vi "RDS Child Subscription.vi"(8 "error in (no error)":errorcluster, 11 "AIP Instrument in":refnum<class "AIP Instrument.lvclass">) -> (0 "error out":errorcluster, 2 "Subscribed IDs":T1[](array[typedef]), 3 "AIP Instrument out":refnum<class "AIP Instrument.lvclass">)   [LabVIEW 2015]
uses:
  Libraries/RDS Framework/RDS Message ID.ctl
  Libraries/RDS Framework/RDS Framework.lvlib
  Actors/RDS Parent Actor/RDS Parent Actor/RDS Parent Actor.lvclass
  AIP Instrument.lvclass
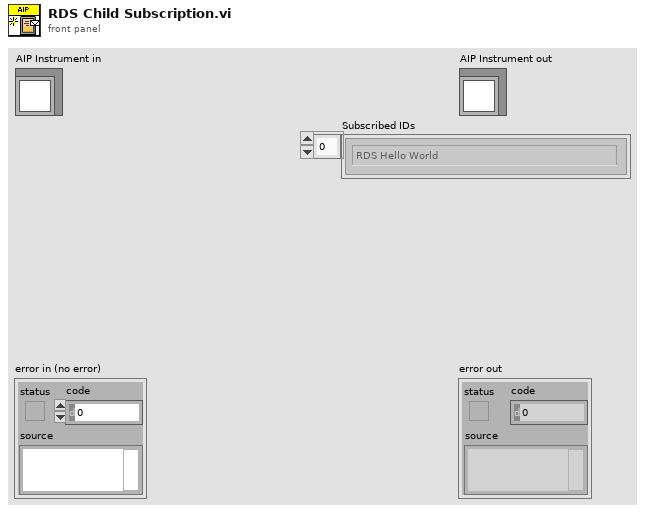
[diagram p1: front panel]
types:
  T1 = typedef "RDS Framework.lvlib/RDS Message ID.ctl" = enum16{"RDS Hello World", "String Message", "AIP_Status", "AIP_Command"}
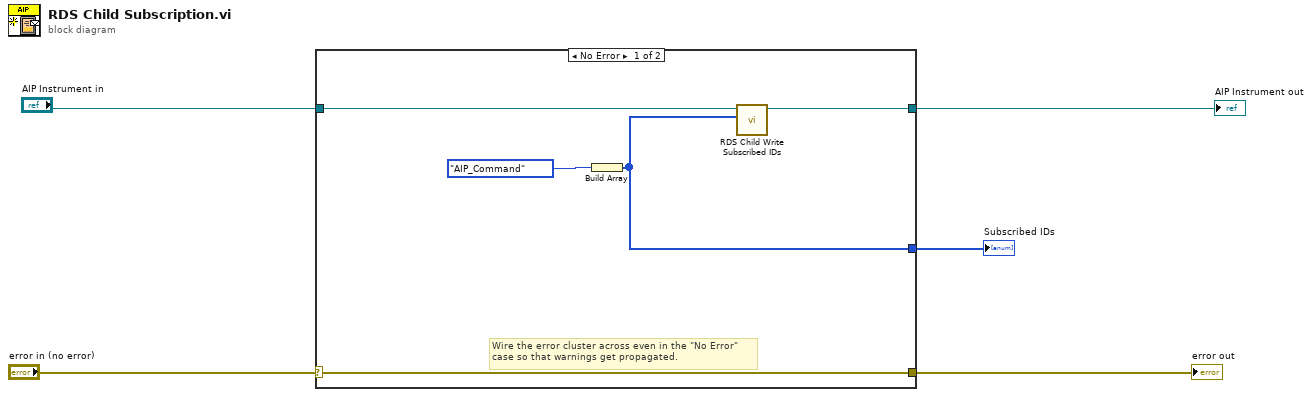
[diagram p0: block diagram]
diagram:
  n1 = case shown="No Error" "error in (no error)" {
    selector: "error in (no error)" -> [w10 w12]
    tunnel: [w10 w12] -> w1
    tunnel: [w7 w11] -> w4
    tunnel: "AIP Instrument in" -> [w8 w11]
    tunnel: [w6 _] -> w5
    frame No Error {
      # "Wire the error cluster across even in the \"No Error\"\ncase so that warnings get propagated."
      n2 = Build Array(RDS_Message_ID."AIP_Command" ("RDS Message")) -> (w6:T1[])
      n3 = call "RDS Child Write Subscribed IDs.vi"("Subscribed IDs"=w6, "RDS Parent Actor in"=w8) -> ("RDS Parent Actor out"=w7:refnum<class "AIP Instrument.lvclass">)  [unwired: 8 in, 1 out]
    }
    frame Error {
    }
  }
  "error out" <- w1
  "AIP Instrument out" <- w4
  "Subscribed IDs" <- w5
